vi "SPI Block Write Read Bytes.vi"(0 "DevHandle":i32, 1 "pReadData":u8[](array[numeric])=array[4097 elements], 2 "BlockNum":i32, 5 "SPIIndex":i32, 7 "pWriteData":u8[](array[numeric])=array[4097 elements], 9 "WriteBlockSize":i32, 12 "ReadBlockSize":i32, 13 "IntervalTimeUs":i32) -> (3 "pReadData out":u8[](array[numeric]), 4 "function return":i32, 8 "pWriteData out":u8[](array[numeric]))   [LabVIEW 2010, in "usb2spi.lvlib"]
doc: "int WINAPI SPI_BlockWriteReadBytes(int DevHandle,int SPIIndex,unsigned char *pWriteData,int WriteBlockSize,unsigned char *pReadData,int ReadBlockSize,int BlockNum,int IntervalTimeUs);"
uses:
  usb2spi.lvlib
  USB2XXX/trunk/USB2XXX/USB2XXX/vs2019/Release/USB2XXX.dll
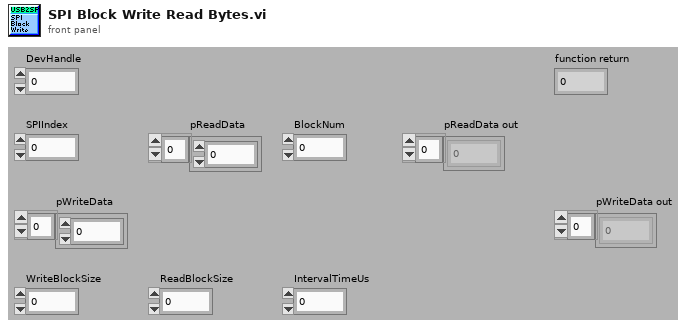
[diagram p1: front panel]
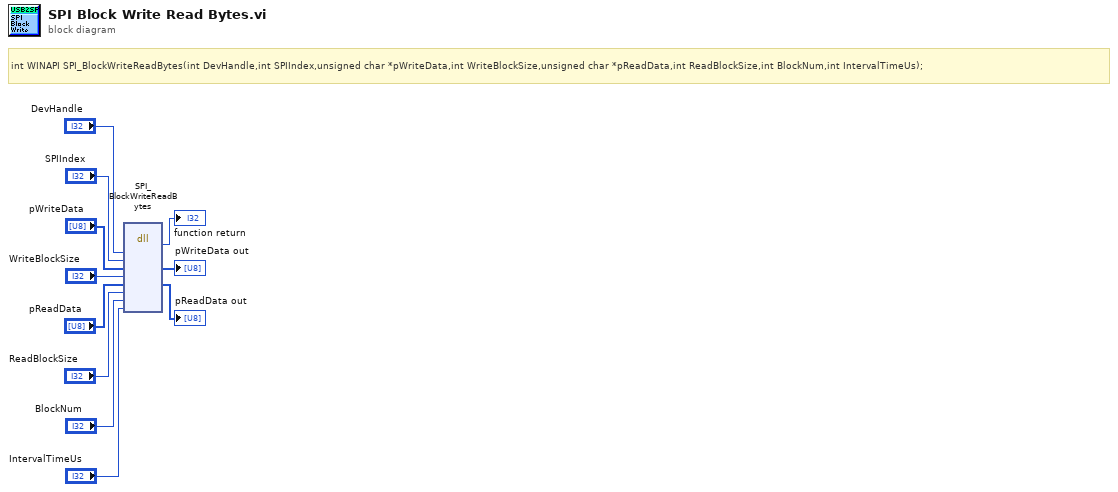
[diagram p0: block diagram]
diagram:
  # "int WINAPI SPI_BlockWriteReadBytes(int DevHandle,int SPIIndex,unsigned char *pWriteData,int WriteBlockSize,unsigned char *pReadData,int ReadBlockSize,int BlockNum,int IntervalTimeUs);"
  n1 = dll-call lib="E:/Projects/USB2XXX/trunk/USB2XXX/USB2XXX/vs2019/Release/USB2XXX.*" fn="SPI_BlockWriteReadBytes"("DevHandle"="DevHandle", "SPIIndex"="SPIIndex", "pWriteData"="pWriteData", "WriteBlockSize"="WriteBlockSize", "pReadData"="pReadData", "ReadBlockSize"="ReadBlockSize", "BlockNum"="BlockNum", "IntervalTimeUs"="IntervalTimeUs") -> (→"function return":i32, "pWriteData"=→"pWriteData out":u8[], "pReadData"=→"pReadData out":u8[])  [unwired: 9 in, 2 out]
